vi "Set Panel State.vi"(10 "Front Panel Window:State":T1(ring), 11 "Base Event in":refnum<class "Base Event.lvclass">) -> (3 "Base Event out":refnum<class "Base Event.lvclass">)   [LabVIEW 2021, in "jettl.lvlib" / "Base Event.lvlib" / "Base Event.lvclass"]
uses:
  Base Event.lvclass
  Base Event.lvclass/Base Event.ctl
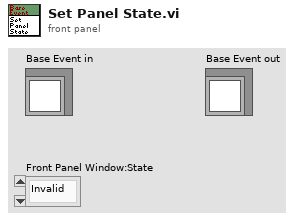
[diagram p1: front panel]
types:
  T1 = enum32{"Invalid", "Standard", "Closed", "Hidden", "Minimized", "Maximized"}
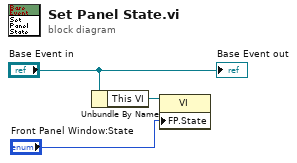
[diagram p0: block diagram]
diagram:
  n1 = Unbundle By Name("Base Event in") -> ("This VI"=w2:refnum<vi>)
  n2 = property class="VI"(reference=w2, "FP.State"="Front Panel Window:State") -> ()  [unwired: 1 in, 2 out]
  "Base Event out" <- "Base Event in"
